vi "IMAQ FPGA Camera Link 4 Tap 8-Bit 4 X-Zones.vi"(6 "Ready for Output":bool=TRUE, 7 "Camera Link Enables":T3, 8 "Cancel Acquisition":bool, 9 "Acquire":bool=TRUE, 10 "Camera Link Data":T2, 11 "Acquisition Settings":T4) -> (0 "Output Valid":bool, 2 "Acquisition Status":T1, 3 "Vision Pixel Bus Out":T5={"Pixel Data"=[0, 0, 0, 0, 0, 0, 0, 0], "DV"=[FALSE, FALSE, FALSE, FALSE, FALSE, FALSE, FALSE, FALSE], "EOL"=FALSE, "EOI"=FALSE, "Data Type"=enum."U8 x 8"}, 5 "Acquisition Overflow":bool)   [LabVIEW 2017]
doc: "Acquires images from a 4 tap (4X-1Y) Camera Link Camera (4 vertical sections). Ensure that this VI is called from a Single Cycle Timed Loop that is running faster than the pixel clock of the camera.\n\nThe <B>Vision Pixel Bus Out</B> can be connected to Vision FPGA algorithms for processing."
uses:
  <vilib>/visionFPGA/Controls/IMAQ FPGA Pixel Bus u8x8.ctl
  <vilib>/visionFPGA/Basics/Camera Link Acquisition/CL Data to Pixels/IMAQ FPGA Camera Link Data to Pixels 4 Tap 8-Bit.vi
  <vilib>/visionFPGA/Basics/Camera Link Acquisition/Line Builder/IMAQ FPGA Camera Link Line Builder (4 Tap U8 4X-1Y).vi
  <vilib>/visionFPGA/Basics/Camera Link Acquisition/Pixel Bus to Vision Pixel Bus/IMAQ FPGA Camera Link Pixel Bus to Vision Pixel Bus U8x8.vi
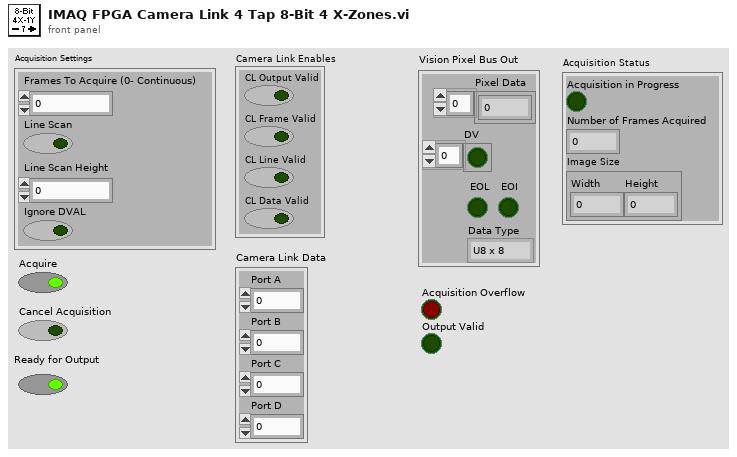
[diagram p1: front panel]
types:
  T1 = cluster{"Acquisition in Progress":bool, "Number of Frames Acquired":u32, "Image Size":cluster{"Width":u32, "Height":u32}}
  T2 = cluster{"Port A":u8, "Port B":u8, "Port C":u8, "Port D":u8}
  T3 = cluster{"CL Output Valid":bool, "CL Frame Valid":bool, "CL Line Valid":bool, "CL Data Valid":bool}
  T4 = cluster{"Frames To Acquire (0- Continuous)":u32, "Line Scan":bool, "Line Scan Height":u32, "Ignore DVAL":bool}
  T5 = typedef "IMAQ FPGA Pixel Bus u8x8.ctl" = cluster{"Pixel Data":u8[], "DV":bool[], "EOL":bool, "EOI":bool, "Data Type":enum16{"U8 x 8"}}
  T6 = cluster{"Acquisition in Progress":bool, "Num Frames Acquired":u32, "Height":u32, "Number of Cycles per Line":u32}
  T7 = cluster{"Acquisition in Progress":bool, "Num Frames Acquired":u32, cluster{u32, "Height":u32}}
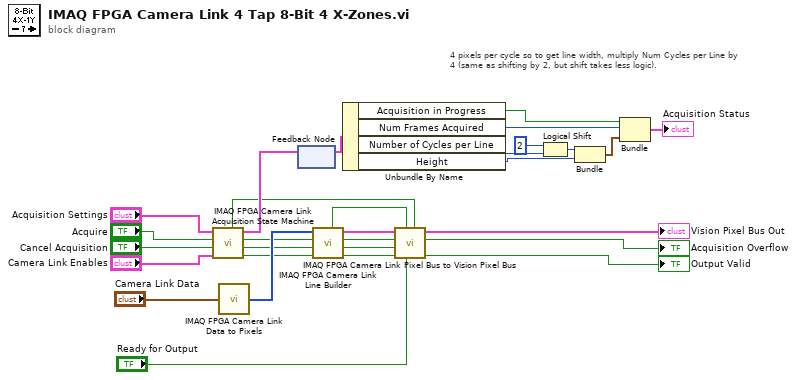
[diagram p0: block diagram]
diagram:
  # "4 pixels per cycle so to get line width, multiply Num Cycles per Line by 4 (same as shifting by 2, but shift takes less logic)."
  n1 = call <vilib>:"IMAQ FPGA Camera Link Acquisition State Machine.vi"("Enables"="Camera Link Enables", "Cancel Acq"="Cancel Acquisition", "Acquire"="Acquire", "Acquisition Settings"="Acquisition Settings") -> ("Output Valid"=w9:bool, "Frame Valid"=w10:bool, "Line Valid"=w11:bool, "Acquisition Status"=w24:T6, "Reset"=w14:bool)  [unwired: 3 in]
  n2 = call-poly <vilib>:"IMAQ FPGA Camera Link Data to Pixels.vi"("Camera Link Data"="Camera Link Data") -> ("Pixels"=w12:u8[])
  n3 = feedback #1() -> (w5:T6)  [unwired: 1 in]
  n4 = feedback-in #1(w24) -> ()
  n5 = call-poly <vilib>:"IMAQ FPGA Camera Link Line Builder.vi"("Input Valid In"=w9, "Frame Valid In"=w10, "Line Valid In"=w11, "Pixel Data In"=w12) -> ("Output Valid"=w26:bool, "Frame Valid Out"=w27:bool, "Line Valid Out"=w28:bool, "Pixel Bus x8 Out"=w29:cluster{"Pixels":u8[], "DV":bool[]}, "Overflow"=w18:bool)  [unwired: 3 in]
  n6 = Unbundle By Name(w5) -> ("Acquisition in Progress"=w3:bool, "Num Frames Acquired"=w4:u32, "Number of Cycles per Line"=w7:u32, "Height"=w25:u32)
  n7 = call-poly <vilib>:"IMAQ FPGA Camera Link Pixel Bus to Vision Pixel Bus.vi"("Reset Overflow"=w14, "Ready for Output"="Ready for Output", "Overflow In"=w18, "Input Valid"=w26, "Frame Valid In"=w27, "Line Valid In"=w28, "Pixel Bus x8 In"=w29) -> ("Output Valid"=→"Output Valid":bool, "Acquisition Overflow"=→"Acquisition Overflow":bool, "Vision Pixel Bus Out"=→"Vision Pixel Bus Out":T5)  [unwired: 2 in]
  n8 = Logical Shift(y=i16 2, x=w7) -> (x << y=w6:u32)
  n9 = Bundle(w6, "Height"=w25) -> (w2:cluster{u32, "Height":u32})  [unwired: 1 in]
  n10 = Bundle("Acquisition in Progress"=w3, "Num Frames Acquired"=w4, w2) -> (→"Acquisition Status":T7)  [unwired: 1 in]
